vi "Scanner Disconnect.vi"(8 "error in (no error)":errorcluster, 11 "Hardware Resources in":T1={"Link"={"Connection"=enum."USB", "Host or IP address (TCP/IP)"="", "Port (Serial/USB)"="COM1"}, "VISA resource"="", "Writer Queue"=refnum, "Status"=FALSE}) -> (0 "error out":errorcluster)   [LabVIEW 2020, in "Hiden Scanner.lvlib"]
doc: "Stops the acquisition."
uses:
  Hiden Scanner.lvlib
  Scanner Hardware Configuration.ctl
  support/Message Queue/Message Cluster.ctl
  <instrlib>/Hiden/Hiden MS.lvlib
  support/Message Queue/Message Queue.lvlib
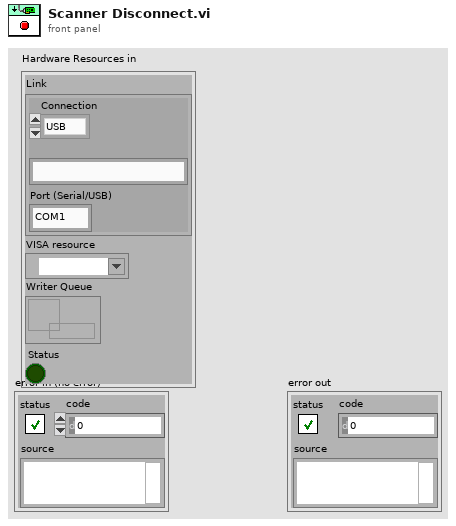
[diagram p1: front panel]
types:
  T1 = typedef "Hiden Scanner.lvlib/Scanner Hardware Configuration.ctl" = cluster{"Link":cluster{"Connection":enum16{"Serial", "TCP/IP", "USB"}, "Host or IP address (TCP/IP)":string, "Port (Serial/USB)":string}, "VISA resource":refnum<visa-resource-name>, "Writer Queue":refnum<queue>, "Status":bool}
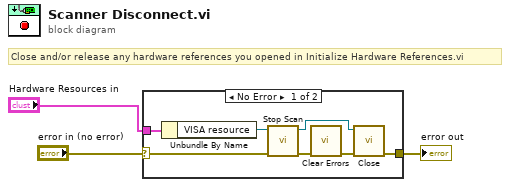
[diagram p0: block diagram]
diagram:
  # "Close and/or release any hardware references you opened in Initialize Hardware References.vi"
  n1 = case shown="No Error" "error in (no error)" {
    selector: "error in (no error)" -> [w5 w11]
    tunnel: [w4 w11] -> w2
    tunnel: "Hardware Resources in" -> [w10 _]
    frame No Error {
      n2 = Unbundle By Name(w10) -> ("VISA resource"=w9:refnum<visa-resource-name>)
      n3 = call <instrlib>:"Stop Scan.vi"("error in (no error)"=w5, "Connection"=w9) -> ("error out"=w7:errorcluster, "Connection (dup)"=w8:refnum<visa-resource-name>)  [unwired: 8 in]
      n4 = call <vilib>:"Clear Errors.vi"("error in (no error)"=w7) -> ("error out"=w6:errorcluster)  [unwired: 5 in, 1 out]
      n5 = call <instrlib>:"Close.vi"("error in (no error)"=w6, "VISA resource name"=w8) -> ("error out"=w4:errorcluster)  [unwired: 9 in]
    }
    frame Error {
    }
  }
  "error out" <- w2
